vi "calibration.vi"() -> ()   [LabVIEW 2019]
uses:
  <vilib>/myRIO/Instrument Drivers/Onboard IO/I2C/typedefs/I2C User Configuration.ctl
  <vilib>/myRIO/Instrument Drivers/Onboard IO/I2C/typedefs/I2C Transfer Rate.ctl
  <vilib>/myRIO/Instrument Drivers/Onboard IO/I2C/typedefs/I2C Reference.ctl
  <vilib>/myRIO/Common/Instrument Driver Framework/Utilities/typedefs/myRIO Generic Hardware Reference.ctl
  <vilib>/myRIO/Common/Instrument Driver Framework/Utilities/typedefs/Hardware Version Enum.ctl
  <vilib>/myRIO/Common/Instrument Driver Framework/Utilities/typedefs/myRIO v1.0 Reference.ctl
  <vilib>/myRIO/Common/Instrument Driver Framework/Utilities/typedefs/Generic FPGA Reference.ctl
  <vilib>/myRIO/Common/Instrument Driver Framework/myRIO v1.0/I2C/typedefs/I2C Channels Enum.ctl
  <vilib>/myRIO/Instrument Drivers/Onboard IO/I2C/typedefs/I2C Configuration.ctl
  <vilib>/userDefined/High Color/nirio_resource_hc.ctl
  <vilib>/Platform/TimedLoop/XDataNode/timing_clust.ctl
  <vilib>/Platform/TimedLoop/XDataNode/nitl_modes.ctl
  <vilib>/Platform/TimedLoop/XDataNode/wakeup.ctl
  <vilib>/myRIO/Common/Instrument Driver Framework/Utilities/vis/Is FPGA Ref Available.vi
  <vilib>/myRIO/Common/Instrument Driver Framework/myRIO v1.0/I2C/vis/myRIO v1.1 Open I2C.vi
  <vilib>/myRIO/Instrument Drivers/Onboard IO/I2C/vis/Configure.vi
  <vilib>/myRIO/Instrument Drivers/Onboard IO/I2C/vis/Write.vi
  <vilib>/myRIO/Instrument Drivers/Onboard IO/I2C/vis/Write Read.vi
  <vilib>/myRIO/Common/Instrument Driver Framework/Utilities/vis/Validate Channels.vi
  <vilib>/myRIO/Common/Instrument Driver Framework/myRIO v1.0/I2C/vis/myRIO v1.0 Reserve I2C.vi
  <vilib>/myRIO/Common/Instrument Driver Framework/myRIO v1.0/UART/vis/myRIO v1.0 Close UART.vi
  <vilib>/myRIO/Common/Instrument Driver Framework/myRIO v1.0/I2C/vis/myRIO v1.0 Build MUX Configuration I2C.vi
  <vilib>/myRIO/Common/Instrument Driver Framework/myRIO v1.0/Resource Manager/vis/myRIO v1.0 Reserve Channel List.vi
  <vilib>/myRIO/Common/Instrument Driver Framework/myRIO v1.0/Resource Manager/vis/myRIO v1.0 Create Configuration List.vi
  <vilib>/myRIO/Common/Instrument Driver Framework/myRIO v1.0/Resource Manager/vis/myRIO v1.0 Reserve Channel.vi
  <vilib>/myRIO/Common/Instrument Driver Framework/myRIO v1.0/Resource Manager/vis/myRIO v1.0 Unreserve Channel.vi
  <vilib>/myRIO/Common/Instrument Driver Framework/myRIO v1.0/Resource Manager/vis/myRIO v1.0 Build Mutex Name.vi
  <vilib>/Utility/VariantDataType/GetNumericInfo.vi
  <vilib>/Utility/error.llb/Error Cluster From Error Code.vi
  <vilib>/myRIO/Common/Instrument Driver Framework/myRIO v1.0/myRIO v1.1 Open.vi
  <vilib>/myRIO/Common/Instrument Driver Framework/Utilities/vis/IO Manager.vi
  <vilib>/myRIO/Common/Instrument Driver Framework/Utilities/vis/Configuration Manager.vi
  <vilib>/myRIO/Common/Instrument Driver Framework/myRIO v1.0/Resource Manager/vis/myRIO v1.0 Configure IO.vi
  <vilib>/myRIO/Common/Instrument Driver Framework/myRIO v1.0/myRIO v1.0 Close.vi
  <vilib>/myRIO/Common/Instrument Driver Framework/myRIO v1.0/I2C/vis/myRIO v1.0 Configure I2C.vi
  <vilib>/myRIO/Common/Instrument Driver Framework/myRIO v1.0/I2C/vis/myRIO v1.0 Write I2C.vi
  <vilib>/Utility/file.llb/Write Delimited Spreadsheet (string).vi
  <vilib>/myRIO/Common/Instrument Driver Framework/myRIO v1.0/I2C/vis/myRIO v1.0 Read I2C.vi
  <vilib>/Utility/file.llb/Write Delimited Spreadsheet (DBL).vi
  <vilib>/myRIO/Common/Instrument Driver Framework/Utilities/vis/FPGA Ref Manager.vi
  <vilib>/myRIO/Common/Instrument Driver Framework/myRIO v1.0/myRIO v1.0 Reset FPGA.vi
  <vilib>/myRIO/Common/Instrument Driver Framework/myRIO v1.0/IRQ/vis/myRIO v1.0 IRQ Info FGV.vi
  <vilib>/myRIO/Common/Instrument Driver Framework/myRIO v1.0/IRQ/vis/myRIO v1.0 Timer IRQ Info FGV.vi
  <vilib>/myRIO/Common/Instrument Driver Framework/myRIO v1.0/IRQ/vis/myRIO v1.0 ISR Agent.vi
  <vilib>/myRIO/Instrument Drivers/Utilities/vis/Reset Index.vi
  <vilib>/myRIO/Common/Instrument Driver Framework/myRIO v1.0/Resource Manager/vis/myRIO v1.0 Block Write Resource Manager.vi
  <vilib>/myRIO/Express VI/Onboard IO/I2C/I2C Express VI.xnode
  <vilib>/myRIO/Instrument Drivers/Onboard IO/I2C/vis/myRIO I2C Open.xnode
  <vilib>/platform/TimedLoop/XDataNode/XDataNode.xnode
  <vilib>/myRIO/Instrument Drivers/Onboard IO/I2C/I2C.lvlib
  <vilib>/Platform/TimedLoop/XDataNode/XDNodeRunTimeDep.lvlib
  <vilib>/myRIO/Instrument Drivers/Utilities/Utilities.lvlib
panel:
  out "Combined Output":cluster{dbl, dbl, dbl, dbl, dbl, dbl}(graph) caption="Waveform Chart"
  out "MUX 2":cluster{dbl, dbl, dbl}(graph) caption="Waveform Chart"
  out "MUX 1":cluster{dbl, dbl, dbl}(graph) caption="Waveform Chart"
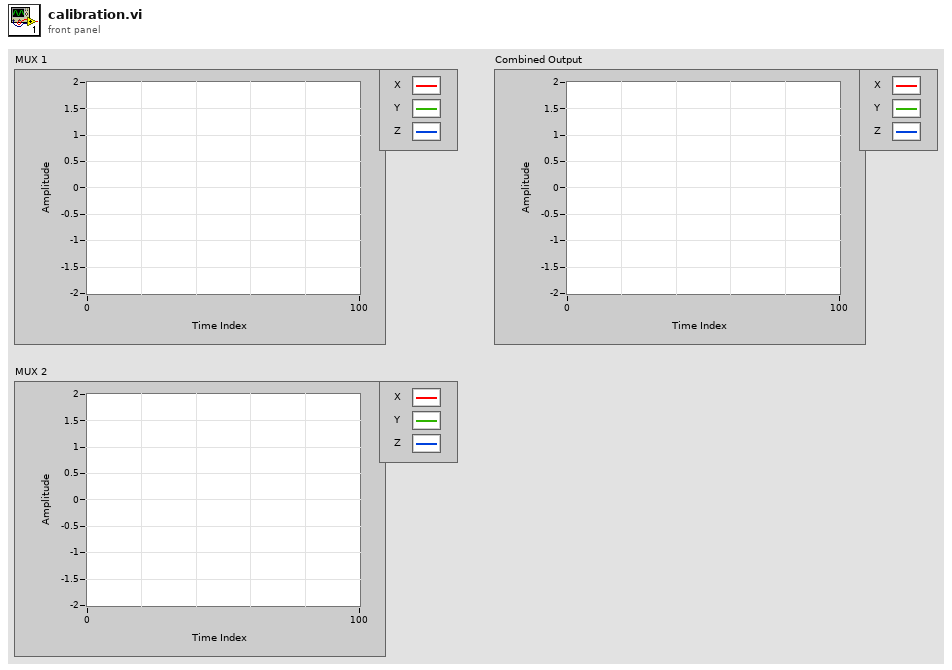
[diagram p1: front panel]
types:
  T1 = typedef "I2C.lvlib/I2C Reference.ctl" = cluster{"myRIO Reference":T2, "I2C Channels Enum":T6, "I2C Configuration":T7}
  T2 = typedef "myRIO Generic Hardware Reference.ctl" = cluster{"myRIO Model":T3, "myRIO Hardware Reference":T4}
  T3 = typedef "Hardware Version Enum.ctl" = enum16{"Unknown", "myRIO-1900", "myRIO-1950", "roboRIO", "NI ELVIS RIO CM", "ELVIS III"}
  T4 = typedef "myRIO v1.0 Reference.ctl" = cluster{"Generic FPGA Reference":T5, "Allow multiple opens":bool}
  T5 = typedef "Generic FPGA Reference.ctl" = refnum<k20>
  T6 = typedef "I2C Channels Enum.ctl" = enum16{"Not Connected", "A/I2C", "B/I2C", "I2C/I2C"}
  T7 = typedef "I2C.lvlib/I2C Configuration.ctl" = cluster{"I2C Transfer Rate":T8}
  T8 = typedef "I2C.lvlib/I2C Transfer Rate.ctl" = enum16{"Standard mode (100 kbps)", "Fast mode (400 kbps)"}
  T9 = typedef "I2C.lvlib/I2C User Configuration.ctl" = cluster{"I2C Transfer Rate":T8}
  T10 = typedef "nirio_resource_hc.ctl" = tag
  T11 = typedef "XDNodeRunTimeDep.lvlib/timing_clust.ctl" = cluster{"Expected End [f-1]":u64, "Actual End [f-1]":u64, "Finished Late? [f-1]":bool, "Expected End [i-1]":u64, "Actual End [i-1]":u64, "Finished Late? [i-1]":bool, "Expected Start [i]":u64, "Actual Start [i]":u64, "Expected Start [f]":u64, "Actual Start [f]":u64, "Source Name":string, "Structure Name":string, "Period":i64, "Deadline":i64, "Offset":i64, "Start":i64, "Priority":i32, "Timeout":i32, "Mode":T12, "Wakeup Reason":T13, "Error":errorcluster, "Source Type":string, "Secondary Source Type":string, "Global End Time":u64, "Global Start Time":u64, "Frame Duration":u64, "Iteration Duration":u64, "Assigned CPU":i32, "I/O Scan Engine Mode":u32}
  T12 = typedef "XDNodeRunTimeDep.lvlib/nitl_modes.ctl" = enum32{"No Change", "Process missed periods, maintain original phase", "Discard missed periods, maintain original phase", "Process missed periods, ignore original phase", "Discard missed periods, ignore original phase"}
  T13 = typedef "XDNodeRunTimeDep.lvlib/wakeup.ctl" = enum32{"Normal", "Aborted", "Asynchronous wakeup", "Timing source error", "Timed loop error", "Timeout"}
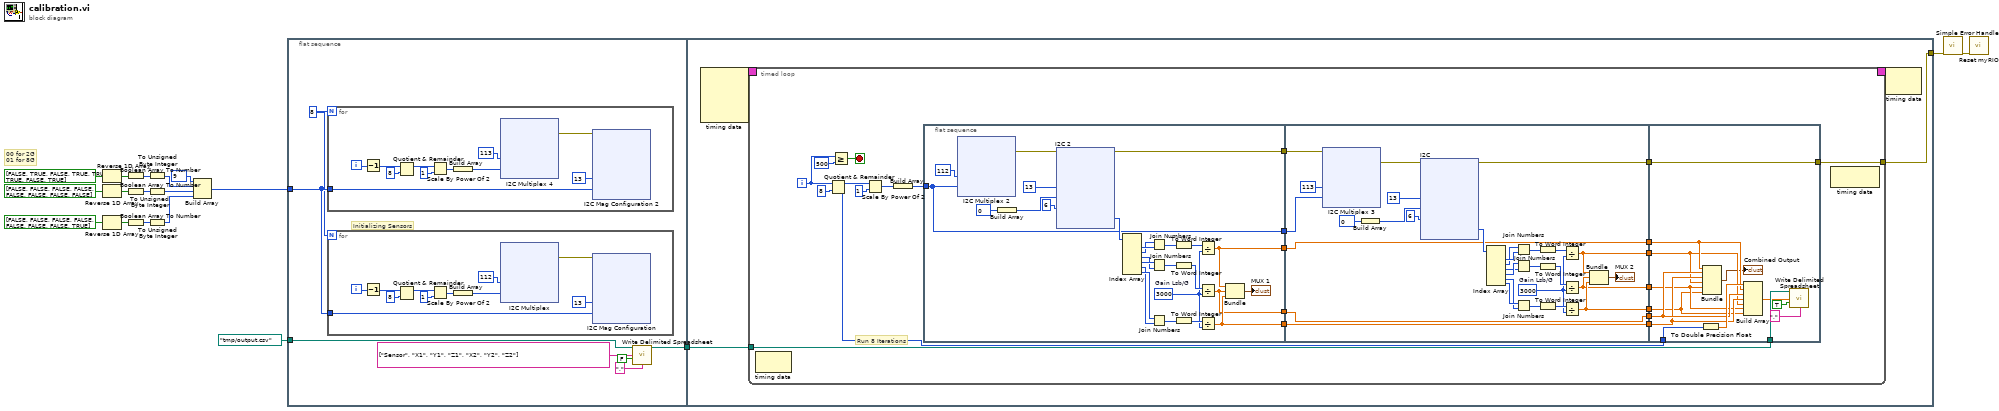
[diagram p0: block diagram]
diagram:
  # "00 for 2G\n01 for 8G"
  n1 = Reverse 1D Array(array=bool[] [FALSE, TRUE, FALSE, TRUE, TRUE, TRUE, FALSE, TRUE]) -> (reversed array=w17:bool[])
  n2 = Reverse 1D Array(array=bool[] [FALSE, FALSE, FALSE, FALSE, FALSE, FALSE, FALSE, FALSE]) -> (reversed array=w16:bool[])
  n3 = Reverse 1D Array(array=bool[] [FALSE, FALSE, FALSE, FALSE, FALSE, FALSE, FALSE, TRUE]) -> (reversed array=w14:bool[])
  n4 = Boolean Array To Number(Boolean array=w17) -> (number=w11:u32)
  n5 = Boolean Array To Number(Boolean array=w16) -> (number=w10:u32)
  n6 = Boolean Array To Number(Boolean array=w14) -> (number=w9:u32)
  n7 = To Unsigned Byte Integer(number=w11) -> (unsigned 8bit integer=w8:u8)
  n8 = To Unsigned Byte Integer(number=w10) -> (unsigned 8bit integer=w7:u8)
  n9 = To Unsigned Byte Integer(number=w9) -> (unsigned 8bit integer=w6:u8)
  n10 = Build Array(u8 9 ("address"), w8, w7, w6) -> (w5:u8[])
  n11 = flat-sequence {
    tunnel: [w25] -> w1
    tunnel: path "/tmp/output.csv" ("file path (dialog if empty)") -> [w21]
    tunnel: w5 -> [w24]
    tunnel: [w200] -> w4
    tunnel: w1 -> [w201]
    frame #0 {
      w23 = 8
      # "Initializing Sensors"
      n12 = for {
        N: w23 -> [_]
        tunnel: w24 -> [w33]
        i -> [w27]
        n13 = Decrement(x=w27) -> (x-1=w26:i32)
        n14 = Quotient & Remainder(x=w26, y=8) -> (x-y*floor(x/y)=w28:i32)  [unwired: 1 out]
        n15 = Scale By Power Of 2(n=w28, x=1) -> (x*2^n=w30:i32)
        n16 = Build Array(w30) -> (w36:i32[])
        n17 = xnode "I2C Multiplex 4"("Slave Address (7-bit)"=u8 113, "Bytes to Write"=w36) -> ("error out"=w35:errorcluster)  [unwired: 1 in]
        n18 = xnode "I2C Mag Configuration 2"("Slave Address (7-bit)"=u8 13, "Bytes to Write"=w33, "error in (no error)"=w35) -> ()  [unwired: 1 out]
      }
      n19 = for {
        N: w23 -> [_]
        tunnel: w24 -> [w120]
        i -> [w114]
        n20 = Decrement(x=w114) -> (x-1=w113:i32)
        n21 = Quotient & Remainder(x=w113, y=8) -> (x-y*floor(x/y)=w115:i32)  [unwired: 1 out]
        n22 = Scale By Power Of 2(n=w115, x=1) -> (x*2^n=w117:i32)
        n23 = Build Array(w117) -> (w123:i32[])
        n24 = xnode "I2C Multiplex"("Slave Address (7-bit)"=u8 112, "Bytes to Write"=w123) -> ("error out"=w122:errorcluster)  [unwired: 1 in]
        n25 = xnode "I2C Mag Configuration"("Slave Address (7-bit)"=u8 13, "Bytes to Write"=w120, "error in (no error)"=w122) -> ()  [unwired: 1 out]
      }
      n26 = call-poly <vilib>:"Write Delimited Spreadsheet.vi"("file path (dialog if empty)"=w21, "1D data"=string[] ["Sensor", "X1", "Y1", "Z1", "X2", "Y2", "Z2"], "append to file? (new file:F)"=FALSE, "delimiter (\\t)"="," ("delimiter (\\t)")) -> ("new file path (Not A Path if cancelled)"=w25:path)  [unwired: 10 in, 1 out]
    }
    frame #1 {
      n27 = node-c288() -> (w203:T11)  [unwired: 4 in]
      n28 = timed-loop {
        timing: w203 -> [_]
        timing-out: [_] -> w202
        tunnel: [w221] -> w200
        tunnel: w201 -> [w204]
        i -> [w206]
        stop <- w205 stop-if-true
        # "Run 8 Iterations"
        n29 = node-c288() -> ()  [unwired: 1 in, 1 out]
        n30 = Quotient & Remainder(x=w206, y=8) -> (x-y*floor(x/y)=w208:i32)  [unwired: 1 out]
        n31 = Greater Or Equal?(x=w206, y=500) -> (x >= y?=w205:bool)
        n32 = Scale By Power Of 2(n=w208, x=1) -> (x*2^n=w209:i32)
        n33 = Build Array(w209) -> (w224:i32[])
        n34 = flat-sequence {
          tunnel: w224 -> [w232]
          tunnel: [w232] -> w222
          tunnel: [w230] -> w220
          tunnel: [w229] -> w214
          tunnel: [w228] -> w212
          tunnel: [w227] -> w210
          tunnel: w222 -> [w340]
          tunnel: w220 -> [w337]
          tunnel: [w338] -> w219
          tunnel: [w336] -> w218
          tunnel: [w335] -> w217
          tunnel: [w334] -> w216
          tunnel: [w333] -> w215
          tunnel: w214 -> [w333]
          tunnel: [w332] -> w213
          tunnel: w212 -> [w332]
          tunnel: [w331] -> w211
          tunnel: w210 -> [w331]
          tunnel: [w451] -> w221
          tunnel: w219 -> [w451]
          tunnel: w218 -> [w442]
          tunnel: w217 -> [w440]
          tunnel: w216 -> [w441]
          tunnel: w215 -> [w443]
          tunnel: w213 -> [w445]
          tunnel: w211 -> [w446]
          tunnel: w208 -> [w450]
          tunnel: w204 -> [w448]
          frame #0 {
            w241 = i16 3000  # Gain Lsb/G
            n35 = xnode "I2C Multiplex 2"("Slave Address (7-bit)"=u8 112, "Bytes to Write"=w232) -> ("error out"=w231:errorcluster)  [unwired: 1 in]
            n36 = Build Array(u8 0) -> (w245:u8[])
            n37 = xnode "I2C 2"("Slave Address (7-bit)"=u8 13, "Bytes to Write"=w245, "Byte Count"=u32 6, "error in (no error)"=w231) -> ("Bytes Read"=w248:u8[], "error out"=w230:errorcluster)
            n38 = Index Array(array=w248) -> (element #1=w240:u8, element #2=w239:u8, element #3=w237:u8, element #4=w238:u8, element #5=w235:u8, element #6=w236:u8)  [unwired: 6 in]
            n39 = Join Numbers(hi=w239, lo=w240) -> ((hi.lo)=w251:u16)
            n40 = Join Numbers(hi=w238, lo=w237) -> ((hi.lo)=w249:u16)
            n41 = Join Numbers(hi=w236, lo=w235) -> ((hi.lo)=w250:u16)
            n42 = To Word Integer(number=w251) -> (16bit integer=w244:i16)
            n43 = To Word Integer(number=w249) -> (16bit integer=w243:i16)
            n44 = To Word Integer(number=w250) -> (16bit integer=w242:i16)
            n45 = Divide(x=w244, y=w241) -> (x/y=w227:dbl)
            n46 = Divide(x=w243, y=w241) -> (x/y=w228:dbl)
            n47 = Divide(x=w242, y=w241) -> (x/y=w229:dbl)
            n48 = Bundle(w227, w228, w229) -> (→"MUX 1":cluster{dbl, dbl, dbl})  [unwired: 1 in]
          }
          frame #1 {
            w349 = i16 3000  # Gain Lsb/G
            n49 = xnode "I2C Multiplex 3"("Slave Address (7-bit)"=u8 113, "Bytes to Write"=w340, "error in (no error)"=w337) -> ("error out"=w339:errorcluster)
            n50 = Build Array(u8 0) -> (w353:u8[])
            n51 = xnode "I2C"("Slave Address (7-bit)"=u8 13, "Bytes to Write"=w353, "Byte Count"=u32 6, "error in (no error)"=w339) -> ("Bytes Read"=w356:u8[], "error out"=w338:errorcluster)
            n52 = Index Array(array=w356) -> (element #1=w348:u8, element #2=w347:u8, element #3=w345:u8, element #4=w346:u8, element #5=w343:u8, element #6=w344:u8)  [unwired: 6 in]
            n53 = Join Numbers(hi=w347, lo=w348) -> ((hi.lo)=w359:u16)
            n54 = Join Numbers(hi=w346, lo=w345) -> ((hi.lo)=w357:u16)
            n55 = Join Numbers(hi=w344, lo=w343) -> ((hi.lo)=w358:u16)
            n56 = To Word Integer(number=w359) -> (16bit integer=w352:i16)
            n57 = To Word Integer(number=w357) -> (16bit integer=w351:i16)
            n58 = To Word Integer(number=w358) -> (16bit integer=w350:i16)
            n59 = Divide(x=w352, y=w349) -> (x/y=w336:dbl)
            n60 = Divide(x=w351, y=w349) -> (x/y=w334:dbl)
            n61 = Divide(x=w350, y=w349) -> (x/y=w335:dbl)
            n62 = Bundle(w336, w334, w335) -> (→"MUX 2":cluster{dbl, dbl, dbl})  [unwired: 1 in]
          }
          frame #2 {
            n63 = To Double Precision Float(number=w450) -> (double precision float=w447:dbl)
            n64 = Bundle(w446, w445, w443, w442, w441, w440) -> (→"Combined Output":cluster{dbl, dbl, dbl, dbl, dbl, dbl})  [unwired: 1 in]
            n65 = Build Array(w447, w446, w445, w443, w442, w441, w440) -> (w439:dbl[])
            n66 = call-poly <vilib>:"Write Delimited Spreadsheet.vi"("file path (dialog if empty)"=w448, "1D data"=w439, "append to file? (new file:F)"=TRUE, "delimiter (\\t)"="," ("delimiter (\\t)")) -> ()  [unwired: 10 in, 2 out]
          }
        }
        n67 = node-c288() -> ()  [unwired: 1 in, 1 out]
      }
      n68 = node-c288(w202) -> ()  [unwired: 1 out]
    }
  }
  n69 = call <vilib>:"Simple Error Handler.vi"("error in (no error)"=w4) -> ("error out"=w3:errorcluster)  [unwired: 4 in, 4 out]
  n70 = call <vilib>:"Reset myRIO.vi"("error in (no error)"=w3) -> ()  [unwired: 10 in, 1 out]
